vi "ErrorHandler.vi"(3 "error in":errorcluster) -> (8 "error?":bool, 11 "error out":errorcluster)   [LabVIEW 2014]
uses:
  phidget21.dll
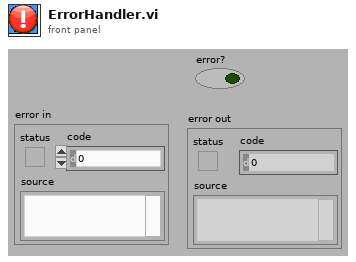
[diagram p1: front panel]
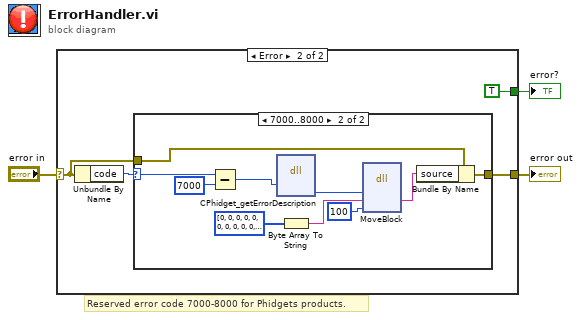
[diagram p0: block diagram]
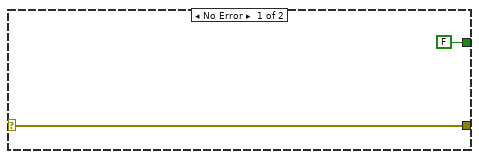
[diagram p2: hidden frame]
diagram:
  # "Reserved error code 7000-8000 for Phidgets products."
  n1 = case shown="Error" "error in" {
    selector: "error in" -> [w5 w9]
    tunnel: [w5 w8] -> w2
    tunnel: [FALSE ("error?") TRUE ("error?")] -> w1
    frame No Error {
    }
    frame Error {
      n2 = Unbundle By Name(w9) -> ("code"=w6:i32)
      n3 = case shown="7000..8000" w6 {
        selector: w6 -> [_ w17]
        tunnel: w9 -> [w10 w20]
        tunnel: [w10 w19] -> w8
        frame 0, Default {
        }
        frame 7000..8000 {
          n4 = Subtract(x=w17, y=7000) -> (x-y=w16:i32)
          n5 = dll-call lib="phidget21.*" fn="CPhidget_getErrorDescription"("ErrorCode"=w16) -> ("ErrorMsg"=w12:i32)  [unwired: 6 in, 2 out]
          n6 = Byte Array To String(unsigned byte array=u8[] [0, 0, 0, 0, 0, 0, 0, 0, 0, 0, 0, 0, 0, 0, 0, 0, 0, 0, 0, 0, 0, 0, 0, 0, 0, 0, 0, 0, 0, 0, 0, 0, 0, 0, 0, 0, 0, 0, 0, 0, 0, 0, 0, 0, 0, 0, 0, 0, 0, 0, 0, 0, 0, 0, 0, 0, 0, 0, 0, 0, 0, 0, 0, 0, 0, 0, 0, 0, 0, 0, 0, 0, 0, 0, 0, 0, 0, 0, 0, 0, 0, 0, 0, 0, 0, 0, 0, 0, 0, 0, 0, 0, 0, 0, 0, 0, 0, 0, 0, 0]) -> (string=w13:string)
          n7 = dll-call lib="LabVIEW" fn="MoveBlock"("pointer"=w12, "string"=w13, "string size"=100) -> ("string"=w11:string)  [unwired: 6 in, 2 out]
          n8 = Bundle By Name(cluster=w20, "source"=w11) -> (w19:errorcluster)
        }
      }
    }
  }
  "error?" <- w1
  "error out" <- w2
